vi "t1.vi"() -> ()   [LabVIEW 2014]
uses:
  <vilib>/FTP/NI_FTP.lvlib
panel:
  in  "숫자형":dbl min=0.0 max=24.0 format="%<%H:%M>t"
  in  "재시작":bool
  in  "2시간":bool
  in  "강제종료":bool
  in  "1시간":bool
  in  "종료취소":bool
  in  "종료":bool
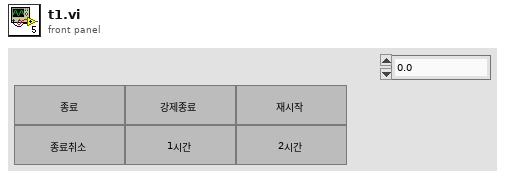
[diagram p1: front panel]
types:
  T1 = typedef "NI_FTP.lvlib/FTP Session.ctl" = refnum<k5>
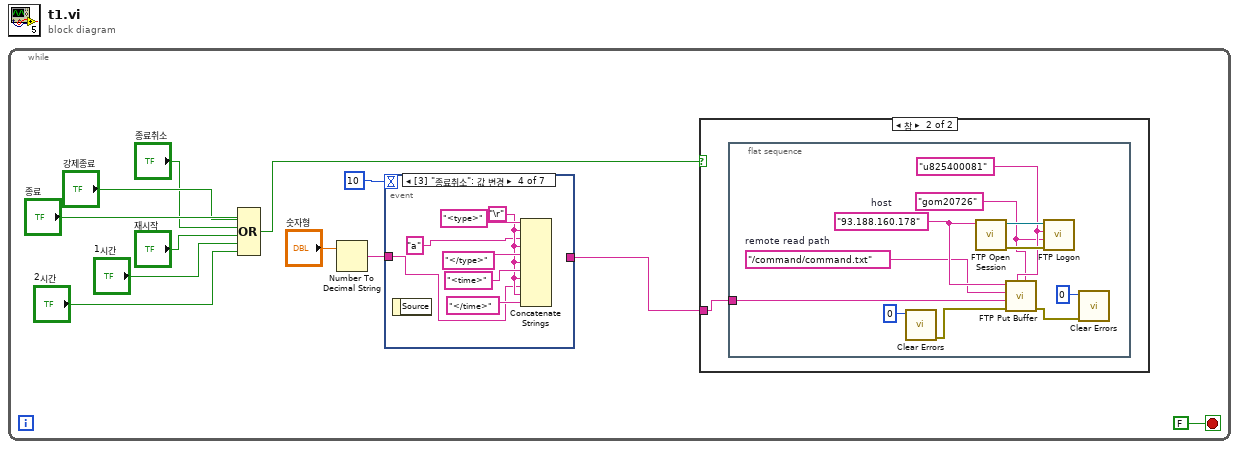
[diagram p0: block diagram]
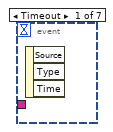
[diagram p3: hidden frame]
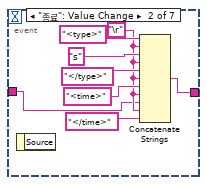
[diagram p4: hidden frame]
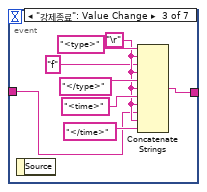
[diagram p5: hidden frame]
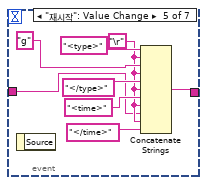
[diagram p6: hidden frame]
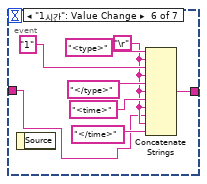
[diagram p7: hidden frame]
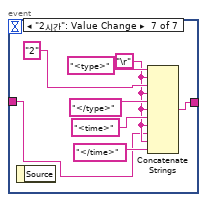
[diagram p8: hidden frame]
diagram:
  n1 = while {
    stop <- FALSE stop-if-true
    n2 = Compound Arithmetic op=OR("종료", "강제종료", "종료취소", "재시작", "1시간", "2시간") -> (w4:bool)
    n3 = Number To Decimal String(number="숫자형") -> (decimal integer string=w11:string)  [unwired: 1 in]
    n4 = event shown="[3] \"종료취소\": 값 변경" {
      selector: _ -> [_ _ _ _ _ _ _]
      dyn-events: _ -> [_ _ _ _ _ _ _]
      timeout: 10 -> [_ _ _ _ _ _ _]
      tunnel: w11 -> [_ w26 w33 w41 w48 w56 w64]
      tunnel: [_ w25 w35 _ w51 w59 w67] -> w2
      event Timeout {
        n5 = event-data() -> ()  [unwired: 1 in, 3 out]
      }
      event "종료": Value Change {
        w27 = "\r"
        n6 = event-data() -> ()  [unwired: 1 in, 1 out]
        n7 = Concatenate Strings("<type>", w27, "s", w27, "</type>", w27, "<time>", w27, w26, w27, "</time>") -> (w25:string)
      }
      event "강제종료": Value Change {
        w36 = "\r"
        n8 = event-data() -> ()  [unwired: 1 in, 1 out]
        n9 = Concatenate Strings("<type>", w36, "f", w36, "</type>", w36, "<time>", w36, w33, w36, "</time>") -> (w35:string)
      }
      event "종료취소": Value Change {
        w43 = "\r"
        n10 = event-data() -> ()  [unwired: 1 in, 1 out]
        n11 = Concatenate Strings("<type>", w43, "a", w43, "</type>", w43, "<time>", w43, w41, w43, "</time>") -> ()  [unwired: 1 out]
      }
      event "재시작": Value Change {
        w49 = "\r"
        n12 = event-data() -> ()  [unwired: 1 in, 1 out]
        n13 = Concatenate Strings("<type>", w49, "g", w49, "</type>", w49, "<time>", w49, w48, w49, "</time>") -> (w51:string)
      }
      event "1시간": Value Change {
        w57 = "\r"
        n14 = event-data() -> ()  [unwired: 1 in, 1 out]
        n15 = Concatenate Strings("<type>", w57, "1", w57, "</type>", w57, "<time>", w57, w56, w57, "</time>") -> (w59:string)
      }
      event "2시간": Value Change {
        w65 = "\r"
        n16 = event-data() -> ()  [unwired: 1 in, 1 out]
        n17 = Concatenate Strings("<type>", w65, "2", w65, "</type>", w65, "<time>", w65, w64, w65, "</time>") -> (w67:string)
      }
    }
    n18 = case shown="참" w4 {
      tunnel: w2 -> [_ w13]
      frame False {
      }
      frame True {
        n19 = flat-sequence {
          tunnel: w13 -> [w18]
          frame #0 {
            w21 = "gom20726"
            w22 = "u825400081"
            w19 = "/command/command.txt"  # remote read path
            w20 = "93.188.160.178"  # host
            n20 = call <vilib>:"Clear Errors.vi"("specific error code to clear (0: all)"=0) -> ("error out"=w16:errorcluster)  [unwired: 5 in, 1 out]
            n21 = call <vilib>:"FTP Open Session.vi"("address"=w20) -> ("error out"=w23:errorcluster, "ftp session"=w24:T1)  [unwired: 7 in, 2 out]
            n22 = call <vilib>:"FTP Put Buffer.vi"("password"=w21, "user"=w22, "error in (no error)"=w16, "data"=w18, "remote path"=w19, "host"=w20) -> ("error out"=w14:errorcluster)  [unwired: 4 in, 1 out]
            n23 = call <vilib>:"FTP Logon.vi"("error in (no error)"=w23, "password"=w21, "user"=w22, "ftp session"=w24) -> ()  [unwired: 4 in, 4 out]
            n24 = call <vilib>:"Clear Errors.vi"("error in (no error)"=w14, "specific error code to clear (0: all)"=0) -> ()  [unwired: 4 in, 2 out]
          }
        }
      }
    }
  }
